vi "Database - Read All Part Numbers.vi"(0 "reference in":refnum<class "Database_UUT.lvclass">, 5 "error in (no error)":errorcluster) -> (14 "reference out":refnum<class "Database_UUT.lvclass">, 18 "group names":string[](array[string]), 19 "error out":errorcluster)   [LabVIEW 2017, in "Database_UUT.lvclass"]
uses:
  Database_UUT.lvclass
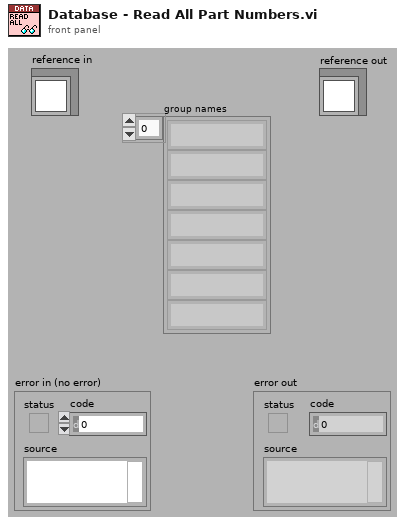
[diagram p1: front panel]
types:
  T1 = enum16{"open", "open or create", "create or replace", "create", "open (read-only)"}
  T2 = typedef "Database_UUT.lvclass/ObjectAttributes.ctl" = cluster{"Filepath to Database":path}
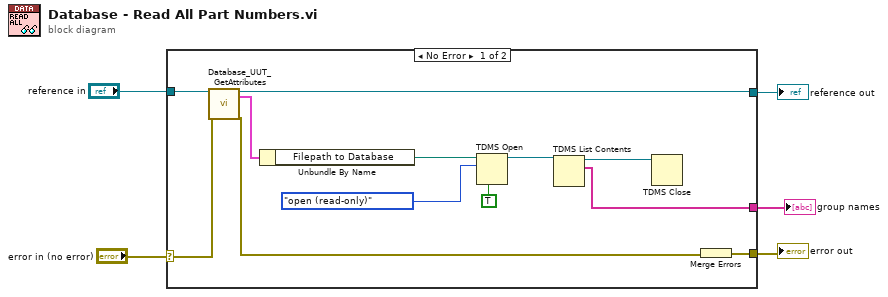
[diagram p0: block diagram]
diagram:
  n1 = case shown="No Error" "error in (no error)" {
    selector: "error in (no error)" -> [w16 w19]
    tunnel: [w12 w19] -> w4
    tunnel: [w14 w18] -> w2
    tunnel: "reference in" -> [w17 w18]
    tunnel: [w6 _] -> w1
    frame No Error {
      n2 = call "Database_UUT_GetAttributes.vi"("reference in"=w17, "error in (no error)"=w16) -> ("reference out"=w14:refnum<class "Database_UUT.lvclass">, "Data"=w15:T2, "error out"=w11:errorcluster)  [unwired: 14 in, 1 out]
      n3 = Unbundle By Name(w15) -> ("Filepath to Database"=w10:path)
      n4 = TDMS Open(6:TRUE ("enable asynchronous? (T)"), 10:T1."open (read-only)" ("operation (0:open)"), 11:w10) -> (3:w8:refnum<k34>)  [unwired: 4 in, 1 out]
      n5 = TDMS List Contents(7:w8) -> (2:w6:string[], 3:w7:refnum<k34>)  [unwired: 2 in, 2 out]
      n6 = TDMS Close(11:w7) -> ()  [unwired: 1 in, 2 out]
      n7 = Merge Errors(w11) -> (w12:errorcluster)
    }
    frame Error {
    }
  }
  "error out" <- w4
  "reference out" <- w2
  "group names" <- w1
